vi "test-trapezoid-profile-switch-goal-in-middle.vi"() -> ()   [LabVIEW 2019]
uses:
  <vilib>/Rock Robotics/WPI/ThirdParty/JAS_Junk/TrajLib/TRAPEZOID_PROFILE_STATE.ctl
  <vilib>/Rock Robotics/WPI/ThirdParty/JAS_Junk/TrajLib/TRAPEZOID_PROFILE.ctl
  <vilib>/Rock Robotics/WPI/ThirdParty/JAS_Junk/TrajLib/TRAPEZOID_PROFILE_CONSTRAINT.ctl
  <vilib>/Rock Robotics/WPI/ThirdParty/JAS_Junk/TrajLib/TrapProfile_ShouldFlipAcceleration.vi
  <vilib>/Rock Robotics/WPI/ThirdParty/JAS_Junk/TrajLib/TrapProfile_Direct.vi
  <vilib>/Rock Robotics/WPI/ThirdParty/JAS_Junk/TrajLib/Trajectory_Library.lvlib
panel:
  out "State 2":T1 {"Velocity" format="%16_6e"; "Position" format="%16_6e"}
  out "Waveform Chart 2":T2(graph)
  out "TRAPEZOID_PROFILE 2":T3 {"Goal"."Velocity" format="%16_6e"; "Goal"."Position" format="%16_6e"; "Initial"."Velocity" format="%16_6e"; "Initial"."Position" format="%16_6e"; "Constraints"."MaxAcceleration" format="%16_6e"; "Constraints"."MaxVelocity" format="%16_6e"; "EndDecel" format="%16_6e"; "EndFullSpeed" format="%16_6e"; "EndAccel" format="%16_6e"}
  out "TRAPEZOID_PROFILE":T3 {"Goal"."Velocity" format="%16_6e"; "Goal"."Position" format="%16_6e"; "Initial"."Velocity" format="%16_6e"; "Initial"."Position" format="%16_6e"; "Constraints"."MaxAcceleration" format="%16_6e"; "Constraints"."MaxVelocity" format="%16_6e"; "EndDecel" format="%16_6e"; "EndFullSpeed" format="%16_6e"; "EndAccel" format="%16_6e"}
  out "State":T1 {"Velocity" format="%16_6e"; "Position" format="%16_6e"}
  out "Waveform Chart":T2(graph)
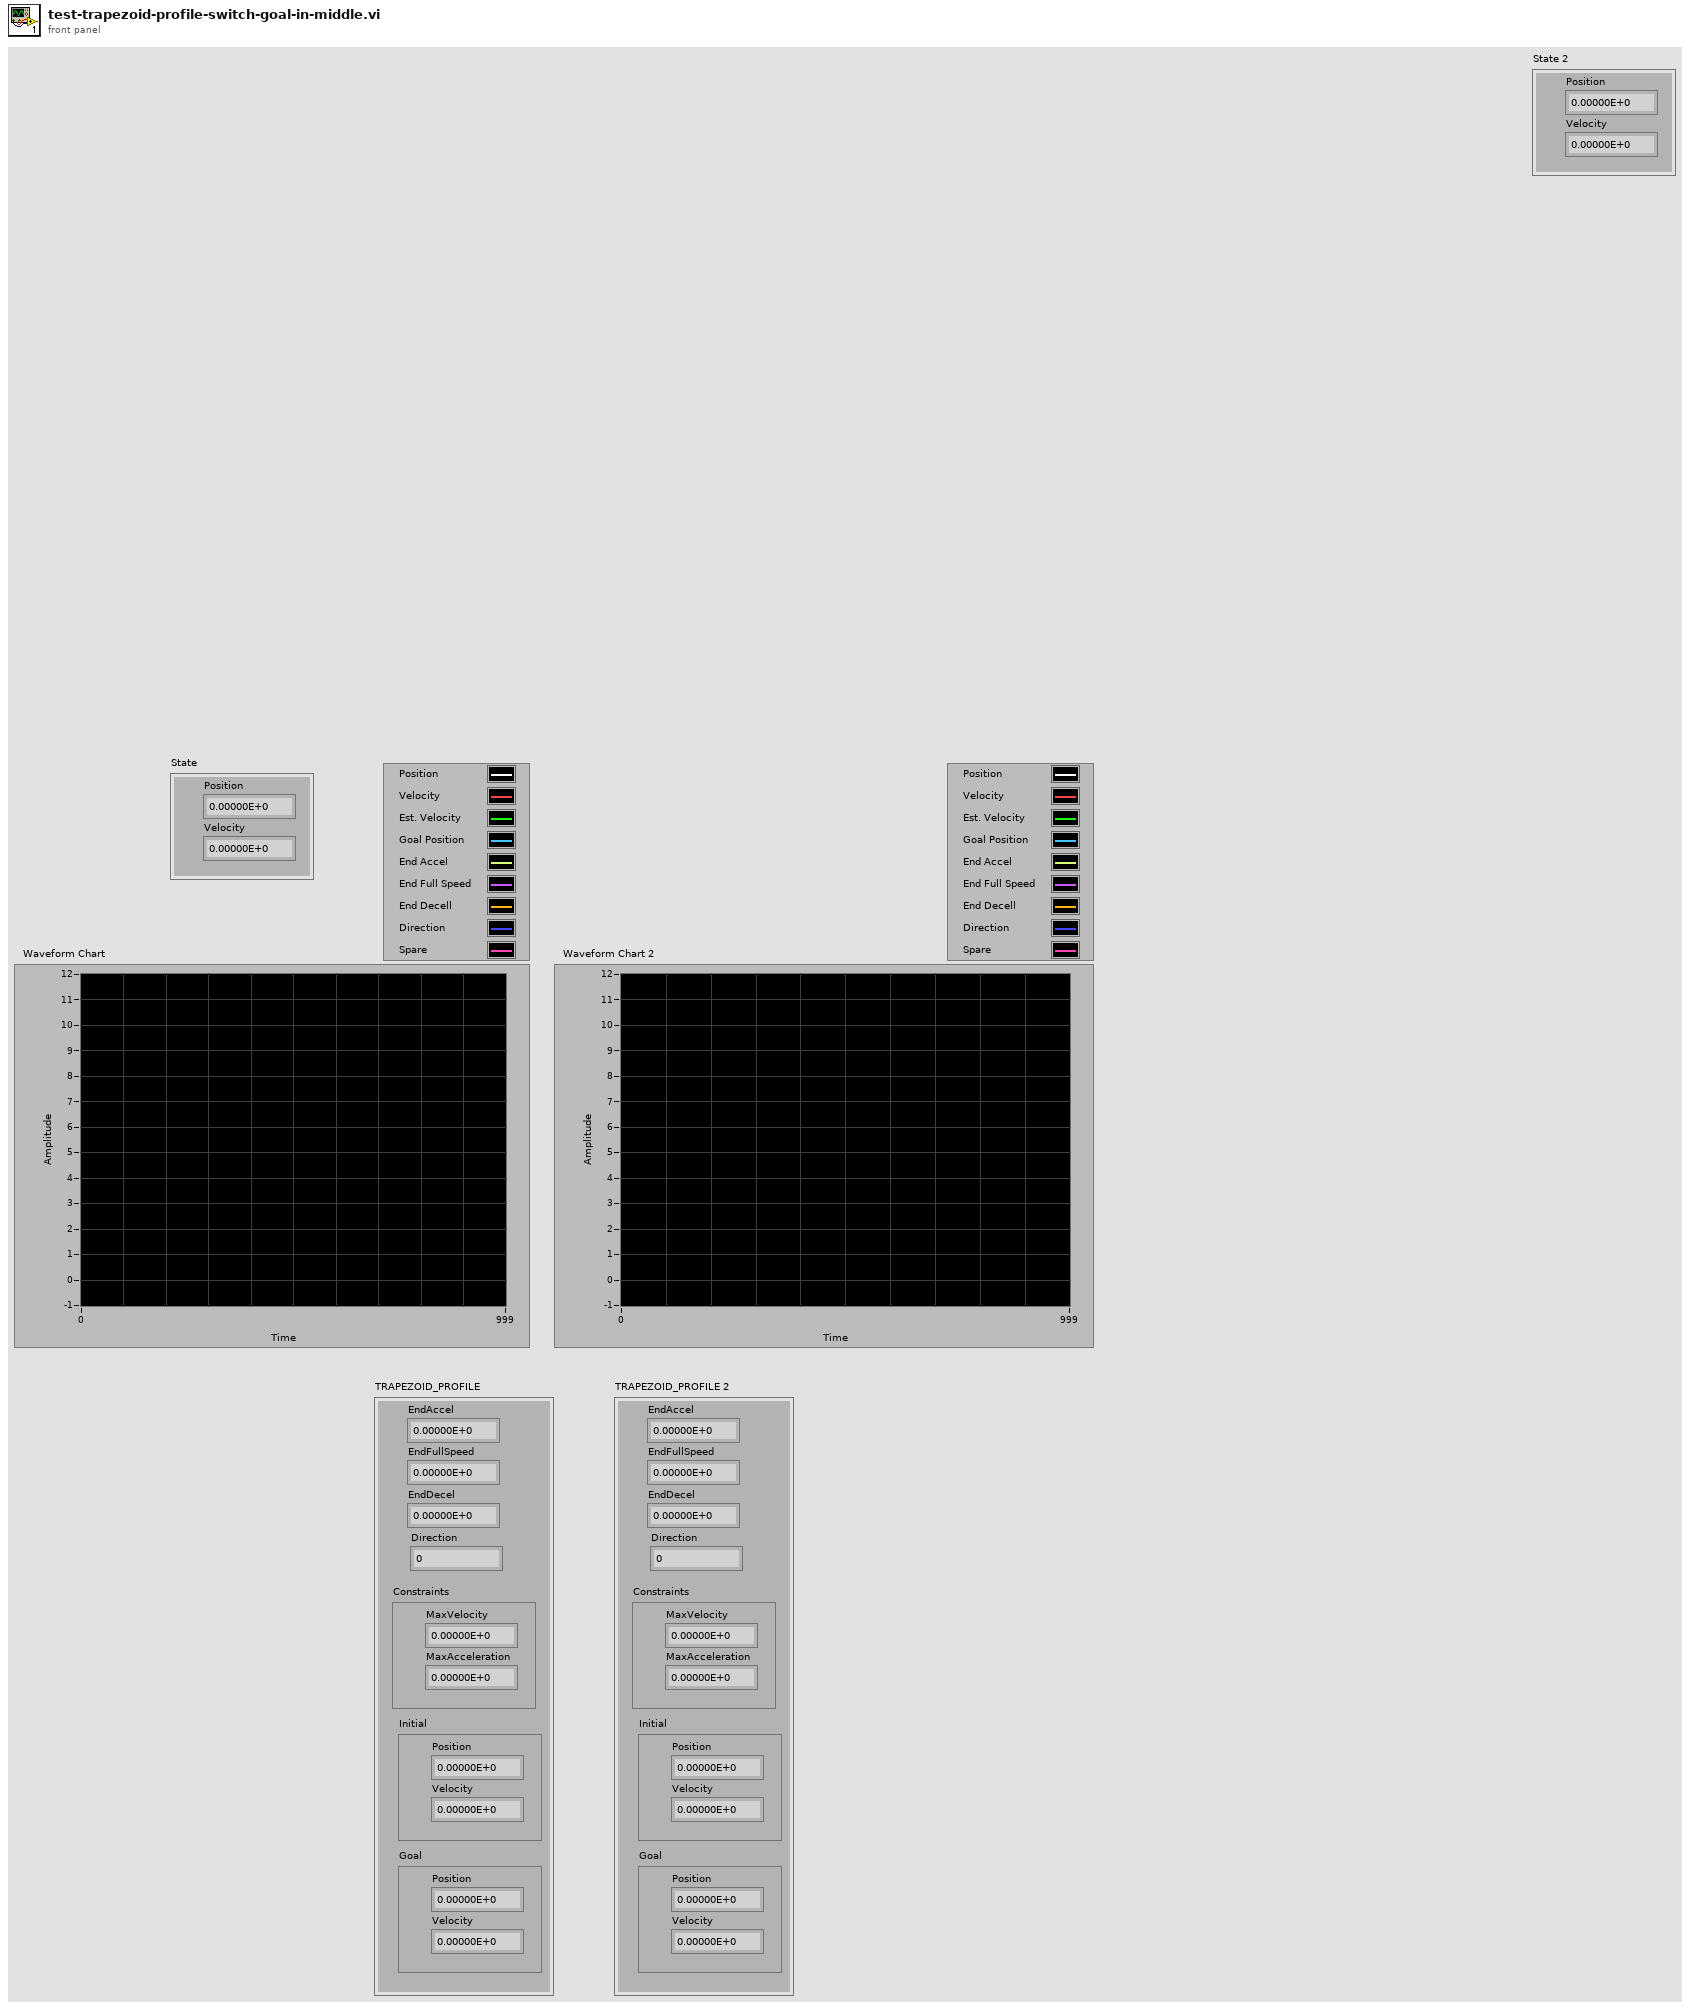
[diagram p1: front panel]
types:
  T1 = typedef "Trajectory_Library.lvlib/TRAPEZOID_PROFILE_STATE.ctl" = cluster{"Position":dbl, "Velocity":dbl}
  T2 = cluster{"Position":dbl, "Velocity":dbl, dbl, "Position":dbl, "EndAccel":dbl, "EndFullSpeed":dbl, "EndDecel":dbl, "Direction":i32, "Position":dbl}
  T3 = typedef "Trajectory_Library.lvlib/TRAPEZOID_PROFILE.ctl" = cluster{"EndAccel":dbl, "EndFullSpeed":dbl, "EndDecel":dbl, "Direction":i32, "Constraints":T4, "Initial":T1, "Goal":T1}
  T4 = typedef "Trajectory_Library.lvlib/TRAPEZOID_PROFILE_CONSTRAINT.ctl" = cluster{"MaxVelocity":dbl, "MaxAcceleration":dbl}
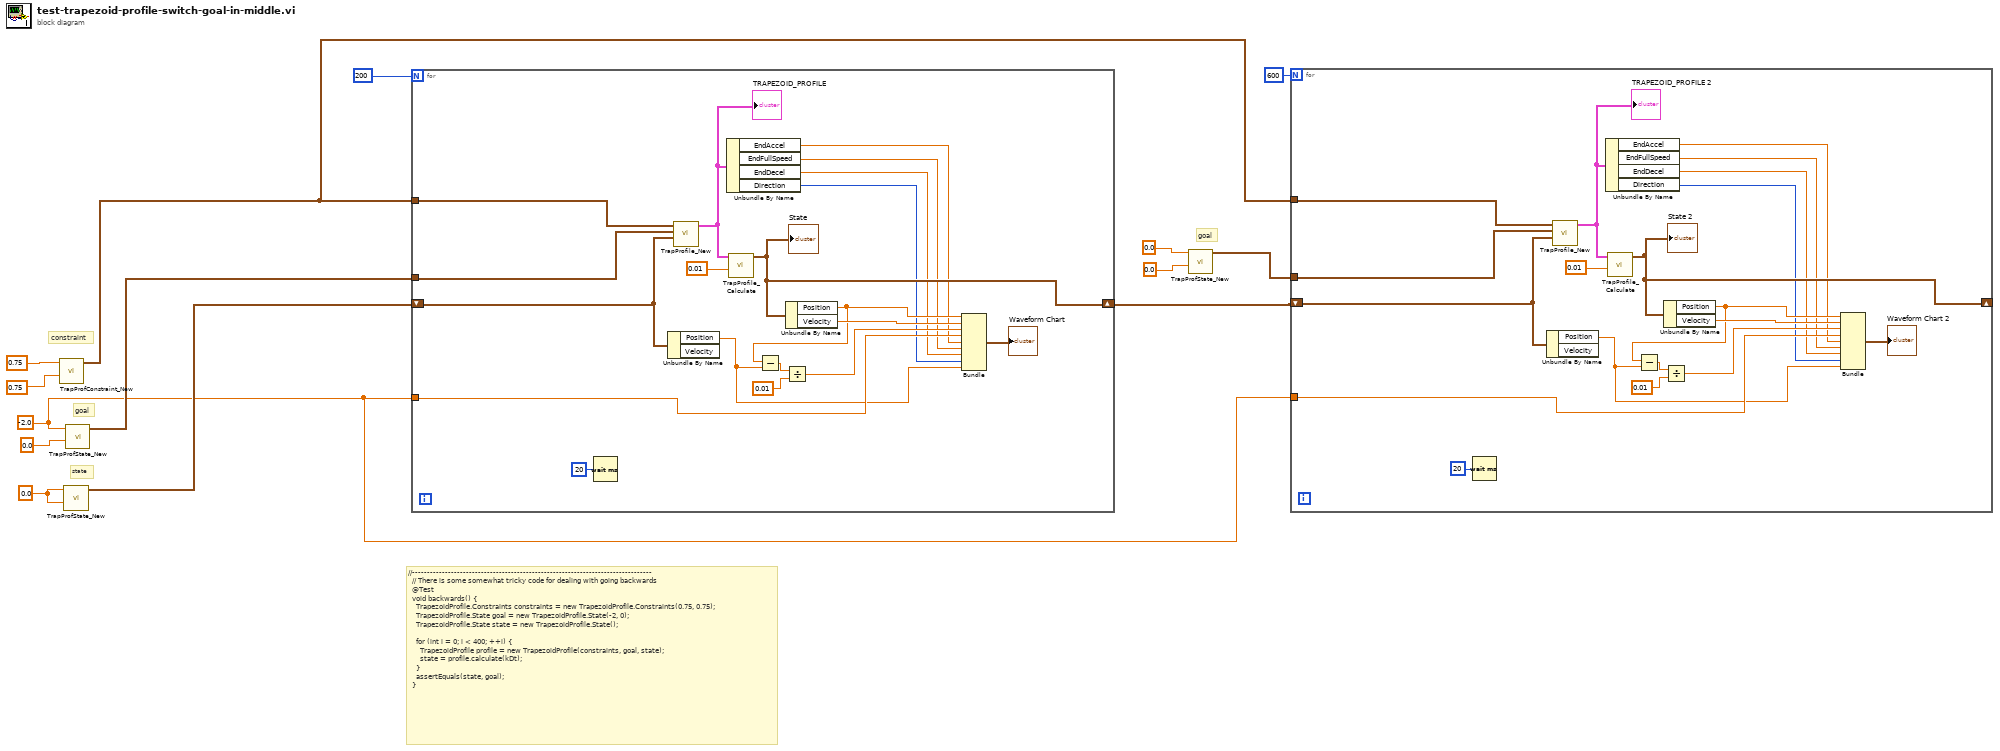
[diagram p0: block diagram]
diagram:
  w9 = 0.0 ("Position")
  w1 = -2.0 ("Position")
  # "goal"
  # "state"
  # "//--------------------------------------------------------------------------------\n  // There is some somewhat tricky code for dealing with going backwards\n  @Test\n  void backwards() {\n    TrapezoidProfile.Constraints constraints = new TrapezoidProfile.Constraints(0.75, 0.75);\n    TrapezoidProfile.State goal = new TrapezoidProfile.State(-2, 0);\n    TrapezoidProfile.State state = new TrapezoidProfile.State();\n\n    for (int i = 0; i < 400; ++i) {\n      TrapezoidProfile profile = new TrapezoidProfile(constraints, goal, state);\n      state = profile.calculate(kDt);\n    }\n    assertEquals(state, goal);\n  }"
  # "goal"
  # "constraint"
  n1 = call <vilib>:"TrapProfConstraint_New.vi"("Max Accel"=0.75, "Max Speed (M/S)"=0.75) -> ("TRAPEZOID_PROFILE_CONSTRAINT"=w2:T4)  [unwired: 9 in]
  n2 = call <vilib>:"TrapProfState_New.vi"("Velocity"=w9, "Position"=w9) -> ("TRAPEZOID_PROFILE_STATE"=w8:T1)  [unwired: 9 in]
  n3 = call <vilib>:"TrapProfState_New.vi"("Velocity"=0.0, "Position"=w1) -> ("TRAPEZOID_PROFILE_STATE"=w10:T1)  [unwired: 9 in]
  n4 = for {
    N: 200 -> [_]
    shift-right: [w23] -> w3
    shift-left: w8 -> [w28]
    tunnel: w10 -> [w30]
    tunnel: w1 -> [w22]
    tunnel: w2 -> [w15]
    n5 = Wait (ms)(milliseconds to wait=u32 20) -> ()  [unwired: 1 out]
    n6 = Unbundle By Name(w28) -> ("Position"=w16:dbl)  [unwired: 1 out]
    n7 = call <vilib>:"TrapProfile_New.vi"("Initial"=w28, "Goal"=w30, "Constraints"=w15) -> ("TRAPEZOID_PROFILE"=w21:T3)  [unwired: 8 in]
    "TRAPEZOID_PROFILE" <- w21
    n8 = Unbundle By Name(w21) -> ("EndAccel"=w20:dbl, "EndFullSpeed"=w19:dbl, "EndDecel"=w18:dbl, "Direction"=w17:i32)
    n9 = call <vilib>:"TrapProfile_Calculate.vi"("Time"=0.01, "TRAPEZOID_PROFILE"=w21) -> ("State"=w23:T1)  [unwired: 9 in]
    "State" <- w23
    n10 = Unbundle By Name(w23) -> ("Position"=w27:dbl, "Velocity"=w31:dbl)
    n11 = Subtract(x=w27, y=w16) -> (x-y=w26:dbl)
    n12 = Divide(x=w26, y=0.01) -> (x/y=w24:dbl)
    n13 = Bundle("Position"=w27, "Velocity"=w31, w24, "Position"=w22, "EndAccel"=w20, "EndFullSpeed"=w19, "EndDecel"=w18, "Direction"=w17, "Position"=w16) -> (→"Waveform Chart":T2)  [unwired: 1 in]
  }
  n14 = call <vilib>:"TrapProfState_New.vi"("Velocity"=0.0, "Position"=0.0) -> ("TRAPEZOID_PROFILE_STATE"=w4:T1)  [unwired: 9 in]
  n15 = for {
    N: 600 -> [_]
    shift-right: [w42] -> _
    shift-left: w3 -> [w47]
    tunnel: w4 -> [w49]
    tunnel: w1 -> [w41]
    tunnel: w2 -> [w34]
    n16 = Wait (ms)(milliseconds to wait=u32 20) -> ()  [unwired: 1 out]
    n17 = Unbundle By Name(w47) -> ("Position"=w35:dbl)  [unwired: 1 out]
    n18 = call <vilib>:"TrapProfile_New.vi"("Initial"=w47, "Goal"=w49, "Constraints"=w34) -> ("TRAPEZOID_PROFILE"=w40:T3)  [unwired: 8 in]
    "TRAPEZOID_PROFILE 2" <- w40
    n19 = Unbundle By Name(w40) -> ("EndAccel"=w39:dbl, "EndFullSpeed"=w38:dbl, "EndDecel"=w37:dbl, "Direction"=w36:i32)
    n20 = call <vilib>:"TrapProfile_Calculate.vi"("Time"=0.01, "TRAPEZOID_PROFILE"=w40) -> ("State"=w42:T1)  [unwired: 9 in]
    "State 2" <- w42
    n21 = Unbundle By Name(w42) -> ("Position"=w46:dbl, "Velocity"=w50:dbl)
    n22 = Subtract(x=w46, y=w35) -> (x-y=w45:dbl)
    n23 = Divide(x=w45, y=0.01) -> (x/y=w43:dbl)
    n24 = Bundle("Position"=w46, "Velocity"=w50, w43, "Position"=w41, "EndAccel"=w39, "EndFullSpeed"=w38, "EndDecel"=w37, "Direction"=w36, "Position"=w35) -> (→"Waveform Chart 2":T2)  [unwired: 1 in]
  }
